vi "Read UDP.vi"(8 "error in (no error)":errorcluster, 11 "Telemetry Server Module in":refnum<class "Telemetry Server Module.lvclass">) -> (0 "error out":errorcluster, 3 "Telemetry Server Module out":refnum<class "Telemetry Server Module.lvclass">)   [LabVIEW 2020, in "Volatus.lvlib" / "Telemetry Server Module.lvclass"]
uses:
  Telemetry Server Module.lvclass
  C:/dev/lv20CE/relink/lv-volatus/Volatus/Module/Module.lvclass
  Module/Module.lvclass/Module.ctl
  Telemetry Server Module.lvclass/Telemetry Server Module.ctl
  IP Endpoint.ctl
  <vilib>/Utility/miscctls.llb/LVMapReplaceAction.ctl
  Event Level.ctl
  lv-vecto/Vecto/proto/UdpPayload/Unflatten.vi
  <vilib>/Utility/error.llb/Error Cluster From Error Code.vi
  lv-vecto/Vecto/Vecto.lvlib
  Module/Module.lvclass
  VolatusAPI/VolatusAPI.lvclass
  Volatus.lvlib
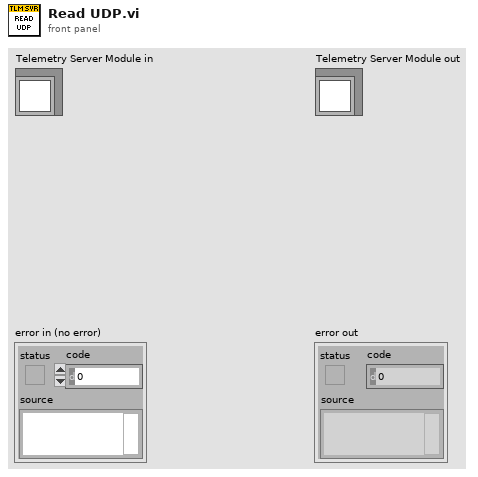
[diagram p1: front panel]
types:
  T1 = typedef "Volatus.lvlib/Telemetry Server Module.lvclass/IP Endpoint.ctl" = cluster{"IP":u32, "Port":u16}
  T2 = typedef "LVMapReplaceAction.ctl" = enum32{"Modify Entry only if found", "Add or Modify Entry", "Delete Entry"}
  T3 = typedef "Volatus.lvlib/Event Level.ctl" = enum16{"Debug", "Info", "Warning", "Error"}
  T4 = typedef "UdpPayload.lvlib/Data.ctl" = cluster{"source_id":u32, "sequence":u32, "timestamp":i64, "type":string, "payload":u8[]}
  T5 = typedef "Volatus.lvlib/Telemetry Server Module.lvclass/Client Info.ctl" = cluster{"Groups":string[], "Last HB":timestamp, "Node ID":u32}
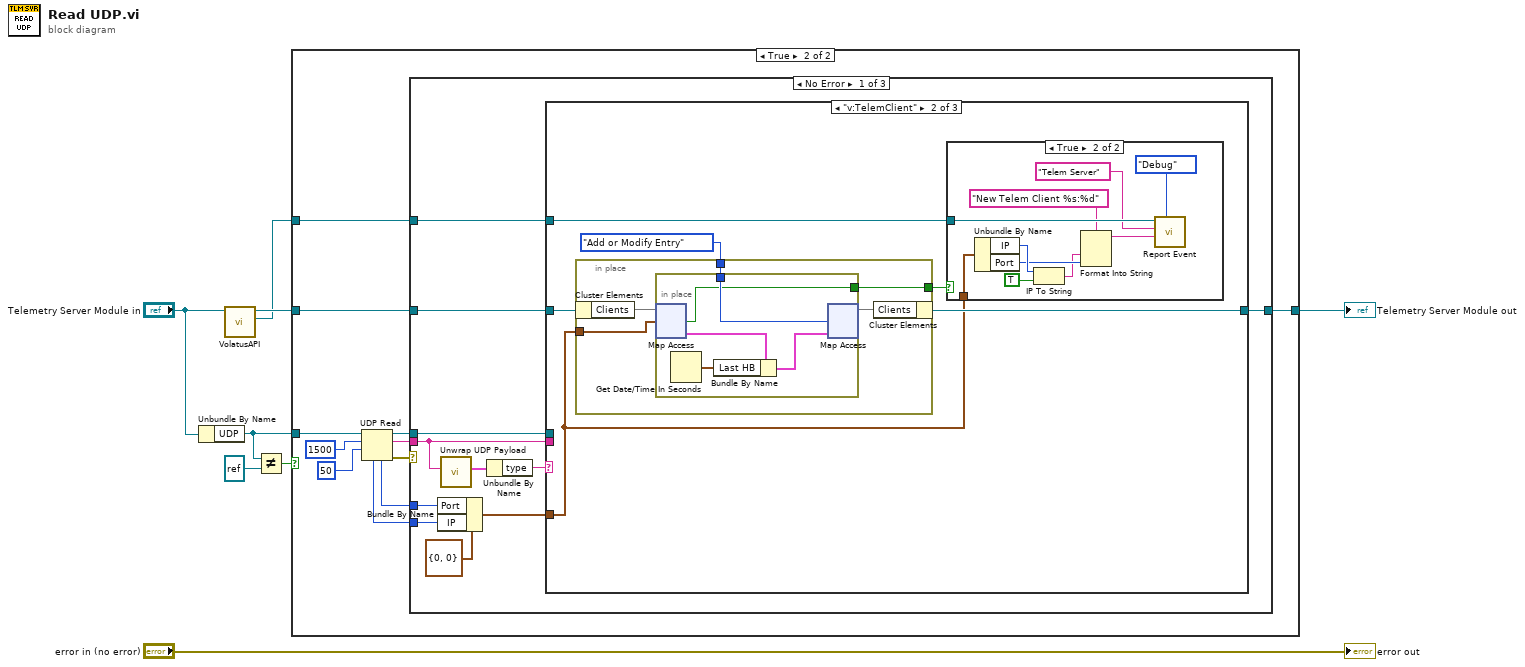
[diagram p0: block diagram]
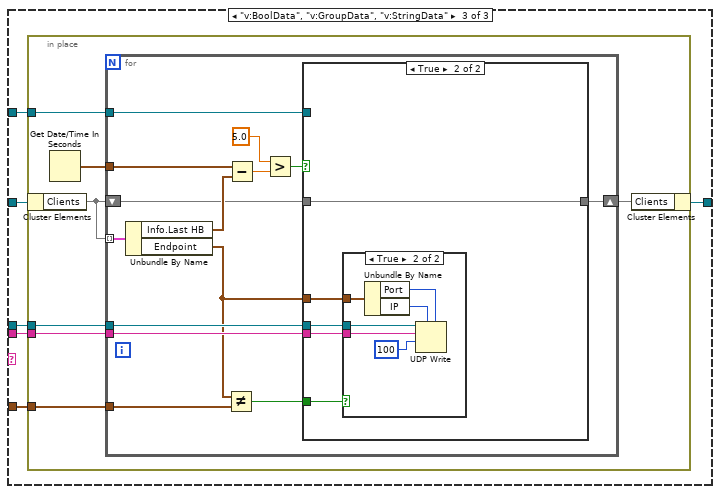
[diagram p5: hidden frame]
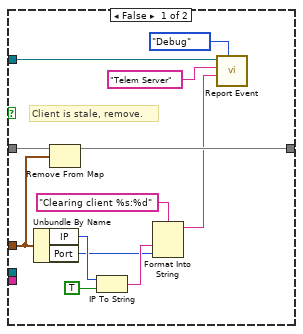
[diagram p6: hidden frame]
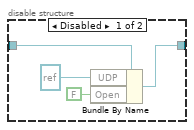
[diagram p9: hidden frame]
diagram:
  n1 = Unbundle By Name("Telemetry Server Module in") -> ("UDP"=w5:refnum<k16>)
  n2 = call "VolatusAPI.vi"("Module in"="Telemetry Server Module in") -> ("VolatusAPI"=w1:refnum<class "VolatusAPI.lvclass">, "Module out"=w2:refnum<class "Telemetry Server Module.lvclass">)  [unwired: 9 in]
  n3 = Not Equal?(x=w5, y=refnum<k16> refnum) -> (x != y?=w6:bool)
  n4 = case shown="True" w6 {
    tunnel: w5 -> [_ w18]
    tunnel: w2 -> [w9 w13]
    tunnel: [w9 w11] -> w4
    tunnel: w1 -> [_ w10]
    frame False {
      # "UDP not open"
    }
    frame True {
      n5 = UDP Read(connection ID=w18, max size (548)=1500, timeout ms (25000)=50) -> (data out=w16:string, error out=w17:errorcluster, 3:w12:refnum<k16>, 4:w14:u16, 6:w15:u32)  [unwired: 1 in]
      n6 = case shown="No Error" w17 {
        tunnel: w16 -> [w26 _ _]
        tunnel: w15 -> [w30 _ _]
        tunnel: w14 -> [w29 _ _]
        tunnel: w13 -> [w25 w110 w116]
        tunnel: w12 -> [w27 _ _]
        tunnel: [w23 w109 w116] -> w11
        tunnel: w10 -> [w21 _ _]
        frame No Error {
          n7 = Bundle By Name(cluster=T1 {"IP"=0, "Port"=0} ("Endpoint"), "Port"=w29, "IP"=w30) -> (w28:T1)
          n8 = call "Unwrap UDP Payload.vi"("UDP Payload"=w26) -> ("Data"=w24:T4)  [unwired: 9 in, 1 out]
          n9 = Unbundle By Name(w24) -> ("type"=w22:string)
          n10 = case shown="\"v:TelemClient\"" w22 {
            tunnel: w28 -> [_ w33 w64]
            tunnel: w27 -> [_ _ w63]
            tunnel: w26 -> [_ _ w62]
            tunnel: w25 -> [w32 w38 w61]
            tunnel: [w32 w37 w60] -> w23
            tunnel: w21 -> [_ w35 w59]
            frame Default {
            }
            frame "v:TelemClient" {
              n11 = in-place {
                in-place-border: w33 -> [w52]
                in-place-border: LVMapReplaceAction."Add or Modify Entry" ("action") -> [w50]
                in-place-border: [w49] -> w34
                n12 = in-place-cluster #1(w38) -> ("Clients"=w53:map{T1, T5})
                n13 = in-place {
                  in-place-border: w50 -> [w55]
                  in-place-border: [w54] -> w49
                  n14 = in-place-map #2(w53, w52) -> (w56:T5, w54:bool)  [unwired: 1 in]
                  n15 = Get Date/Time In Seconds() -> (seconds since 1Jan1904=w57:timestamp)
                  n16 = Bundle By Name(cluster=w56, "Last HB"=w57) -> (w58:T5)
                  n17 = in-place-map #2(w58, w55) -> (w51:map{T1, T5})  [unwired: 2 out]
                }
                n18 = in-place-cluster #1("Clients"=w51) -> (w37:refnum<class "Telemetry Server Module.lvclass">)
              }
              n19 = case shown="True" w34 {
                tunnel: w35 -> [_ w48]
                tunnel: w33 -> [_ w45]
                frame False {
                }
                frame True {
                  n20 = Unbundle By Name(w45) -> ("IP"=w44:u32, "Port"=w42:u16)
                  n21 = IP To String(1:TRUE ("dot notation? (F)"), 2:w44) -> (0:w41:string)
                  n22 = Format Into String(format string="New Telem Client %s:%d", w41, w42) -> (resulting string=w40:string)  [unwired: 2 in, 1 out]
                  n23 = call "Report Event.vi"("Level (Info)"=Event_Level."Debug", "Message"=w40, "Context"="Telem Server", "VolatusAPI in"=w48) -> ()  [unwired: 6 in, 2 out]
                }
              }
            }
            frame "v:BoolData", "v:GroupData", "v:StringData" {
              n24 = in-place {
                in-place-border: w64 -> [w71]
                in-place-border: w63 -> [w70]
                in-place-border: w62 -> [w69]
                in-place-border: w59 -> [w65]
                n25 = in-place-cluster #3(w61) -> ("Clients"=w68:map{T1, T5})
                n26 = Get Date/Time In Seconds() -> (seconds since 1Jan1904=w66:timestamp)
                n27 = for {
                  tunnel: w71 -> [w85]
                  tunnel: w70 -> [w84]
                  tunnel: w69 -> [w83]
                  shift-right: [w73] -> w67
                  shift-left: w68 -> [w74]
                  tunnel: w68 -> [w81] mode=indexing
                  tunnel: w66 -> [w79]
                  tunnel: w65 -> [w72]
                  n28 = Unbundle By Name(w81) -> ("Info.Last HB"=w78:timestamp, "Endpoint"=w80:T1)
                  n29 = Not Equal?(x=w80, y=w85) -> (x != y?=w82:bool)
                  n30 = Subtract(x=w79, y=w78) -> (x-y=w77:dbl)
                  n31 = Greater?(x=5.0, y=w77) -> (0:w75:bool)
                  n32 = case shown="True" w75 {
                    tunnel: w84 -> [_ w102]
                    tunnel: w83 -> [_ w101]
                    tunnel: w82 -> [_ w100]
                    tunnel: w80 -> [w95 w99]
                    tunnel: w74 -> [w97 w98]
                    tunnel: [w96 w98] -> w73
                    tunnel: w72 -> [w89 _]
                    frame False {
                      # "Client is stale, remove."
                      n33 = Unbundle By Name(w95) -> ("IP"=w94:u32, "Port"=w90:u16)
                      n34 = Remove From Map(10:w95, 11:w97) -> (3:w96:map{T1, T5})  [unwired: 2 out]
                      n35 = IP To String(1:TRUE ("dot notation? (F)"), 2:w94) -> (0:w91:string)
                      n36 = Format Into String(format string="Clearing client %s:%d", w91, w90) -> (resulting string=w87:string)  [unwired: 2 in, 1 out]
                      n37 = call "Report Event.vi"("Level (Info)"=Event_Level."Debug", "Message"=w87, "Context"="Telem Server", "VolatusAPI in"=w89) -> ()  [unwired: 6 in, 2 out]
                    }
                    frame True {
                      n38 = case shown="True" w100 {
                        tunnel: w102 -> [_ w108]
                        tunnel: w99 -> [_ w107]
                        tunnel: w101 -> [_ w104]
                        frame False {
                        }
                        frame True {
                          n39 = Unbundle By Name(w107) -> ("Port"=w105:u16, "IP"=w106:u32)
                          n40 = UDP Write(address=w106, port or service name=w105, connection ID=w108, data in=w104, 9:100 ("timeout ms (25000)")) -> ()  [unwired: 1 in, 2 out]
                        }
                      }
                    }
                  }
                }
                n41 = in-place-cluster #3("Clients"=w67) -> (w60:refnum<class "Telemetry Server Module.lvclass">)
              }
            }
          }
        }
        frame Default {
          n42 = disable-structure shown="Enabled" {
            disable-tunnel: w110 -> [w114 w115]
            disable-tunnel: [w113 w115] -> w109
            frame Disabled {
              n43 = Bundle By Name(cluster=w114, "UDP"=refnum<k16> refnum, "Open"=FALSE) -> (w113:refnum<class "Telemetry Server Module.lvclass">)
            }
            frame Enabled {
            }
          }
        }
        frame Error {
        }
      }
    }
  }
  "Telemetry Server Module out" <- w4
  "error out" <- "error in (no error)"
